vi "Кластеры-02-функции.vi"() -> ()   [LabVIEW 2017]
panel:
  in  "Boolean":bool
  out "Cluster 2":T1
  in  "Cluster":T2
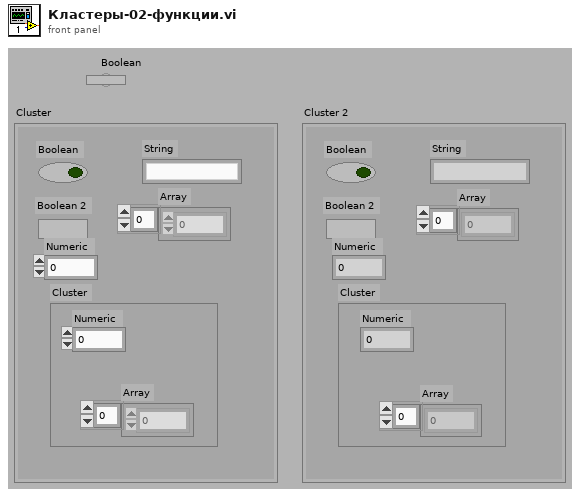
[diagram p1: front panel]
types:
  T1 = cluster{"Array":dbl[], "Cluster":cluster{"Array":u8[], "Numeric":i32}, "Numeric":dbl, "Boolean 2":bool, "String":string, "Boolean":bool}
  T2 = cluster{"Boolean":bool, "Boolean 2":bool, "Numeric":dbl, "String":string, "Array":dbl[], "Cluster":cluster{"Numeric":i32, "Array":u8[]}}
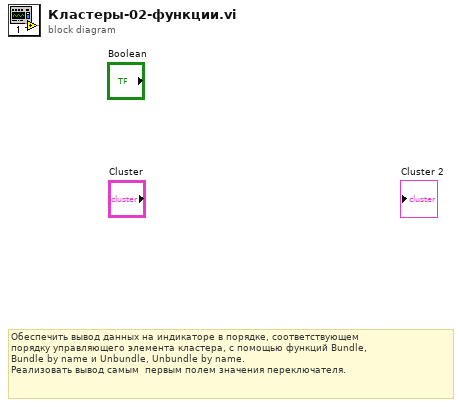
[diagram p0: block diagram]
diagram:
  # "Обеспечить вывод данных на индикаторе в порядке, соответствующем\nпорядку управляющего элемента кластера, с помощью функций Bundle, \nBundle by name и Unbundle, Unbundle by name.\nРеализовать вывод самым  первым полем значения переключателя."
